vi "test Parse Sorted Object Dictionary_2.vi"(11 "Test Case In":refnum<class "test Electronic Datasheet.lvclass">) -> (0 "error out":errorcluster, 3 "Test Case Out":refnum<class "test Electronic Datasheet.lvclass">)   [LabVIEW 2024, in "test Electronic Datasheet.lvclass"]
uses:
  test Electronic Datasheet.lvclass
  C:/Program Files/National Instruments/LabVIEW 2024/vi.lib/Astemes/LUnit/Test Case.lvclass
  Core/Object Type.ctl
  Core/Access Type.ctl
  <vilib>/Astemes/LUnit/Test Case.lvclass/Test Case.ctl
  <vilib>/Astemes/LUnit/Append Fail Result.vi
  <vilib>/Astemes/LUnit/Append Pass Result.vi
  <vilib>/Astemes/LUnit/Run In UI.vi
  <vilib>/Utility/error.llb/Clear Errors.vi
  Core/OD Sub-Entry/OD Sub-Entry.lvclass
  D:/git/EDS-File-Viewer/Core/OD Entry/OD Entry.lvclass
  Electronic Datasheet/utils/Electronic Datasheet_GetAttributes.vi
  test Electronic Datasheet.lvclass/test Electronic Datasheet.ctl
  Electronic Datasheet/Electronic Datasheet.lvclass
  <vilib>/Astemes/LUnit/Test Case.lvclass
  Core/Electronic Datasheet.lvlib
  Core/OD Entry/OD Entry.lvclass
  D:/git/EDS-File-Viewer/Core/OD Sub-Entry/OD Sub-Entry.lvclass
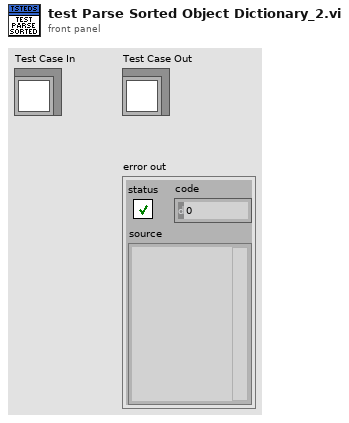
[diagram p1: front panel]
types:
  T1 = typedef "Electronic Datasheet.lvlib/Access Type.ctl" = enum16{"ro", "wo", "rw", "rwr", "rww", "const"}
  T2 = typedef "Electronic Datasheet.lvlib/Object Type.ctl" = u8
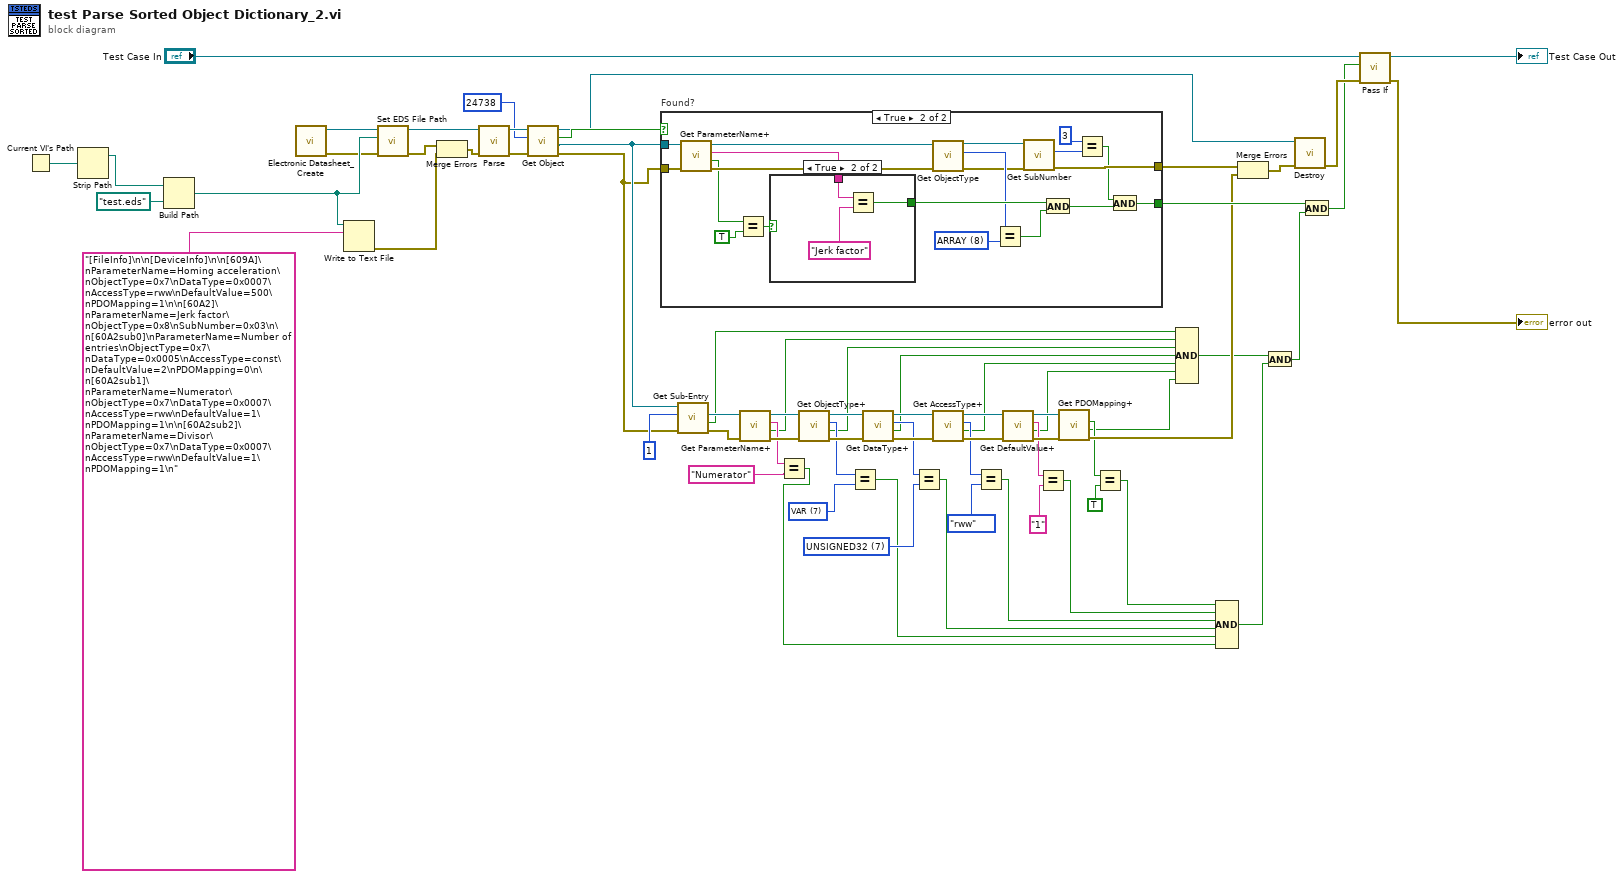
[diagram p0: block diagram]
diagram:
  w37 = u16 7 items=["BOOLEAN"=1, "INTEGER8"=2, "INTEGER16"=3, "INTEGER32"=4, "UNSIGNED8"=5, "UNSIGNED16"=6, "UNSIGNED32"=7, "REAL32"=8, "VISIBLE_STRING"=9, "OCTET_STRING"=10, "UNICODE_STRING"=11, "TIME_OF_DAY"=12, "TIME_DIFFERENCE"=13, "RESERVED1"=14, "DOMAIN"=15, "INTEGER24"=16, "REAL64"=17, "INTEGER40"=18, "INTEGER48"=19, "INTEGER56"=20, "INTEGER64"=21, "UNSIGNED24"=22, "RESERVED2"=23, "UNSIGNED40"=24, "UNSIGNED48"=25, "UNSIGNED56"=26, "UNSIGNED64"=27, "RESERVED3"=28, "RESERVED4"=29, "RESERVED5"=30, "RESERVED6"=31, "PDO_COMMUNICATION_PARAMETER"=32, "PDO_MAPPING"=33, "SDO_PARAMETER"=34, "IDENTITY"=35, "RESERVED7"=36] ("DataType")
  w39 = T2 7 items=["NULL"=0, "DOMAIN"=2, "DEFTYPE"=5, "DEFSTRUCT"=6, "VAR"=7, "ARRAY"=8, "RECORD"=9] ("ObjectType")
  n1 = Current VI's Path() -> (path=w64:path)
  n2 = Strip Path(path=w64) -> (stripped path=w60:path)  [unwired: 1 out]
  n3 = Build Path(base path=w60, name or relative path=path "test.eds") -> (appended path=w61:path)
  n4 = call "Electronic Datasheet_Create.vi"() -> ("Error Out"=w9:errorcluster, "reference out"=w10:refnum<class "Electronic Datasheet.lvclass">)  [unwired: 10 in]
  n5 = Write to Text File(file (use dialog)=w61, text="[FileInfo]\n\n[DeviceInfo]\n\n[609A]\nParameterName=Homing acceleration\nObjectType=0x7\nDataType=0x0007\nAccessType=rww\nDefaultValue=500\nPDOMapping=1\n\n[60A2]\nParameterName=Jerk factor\nObjectType=0x8\nSubNumber=0x03\n\n[60A2sub0]\nParameterName=Number of entries\nObjectType=0x7\nDataType=0x0005\nAccessType=const\nDefaultValue=2\nPDOMapping=0\n\n[60A2sub1]\nParameterName=Numerator\nObjectType=0x7\nDataType=0x0007\nAccessType=rww\nDefaultValue=1\nPDOMapping=1\n\n[60A2sub2]\nParameterName=Divisor\nObjectType=0x7\nDataType=0x0007\nAccessType=rww\nDefaultValue=1\nPDOMapping=1\n") -> (error out=w62:errorcluster)  [unwired: 2 in, 2 out]
  n6 = call "Set EDS File Path.vi"("error in"=w9, "EDS File Path"=w61, "reference in"=w10) -> ("error out"=w1:errorcluster, "reference out"=w65:refnum<class "Electronic Datasheet.lvclass">)  [unwired: 7 in]
  n7 = Merge Errors(w1, w62) -> (w2:errorcluster)
  n8 = call "Parse.vi"("error in"=w2, "reference in"=w65) -> ("error out"=w8:errorcluster, "reference out"=w59:refnum<class "Electronic Datasheet.lvclass">)  [unwired: 8 in]
  n9 = call "Get Object.vi"("error in"=w8, "Index"=u16 24738 ("Numeric"), "reference in"=w59) -> ("error out"=w4:errorcluster, "OD Entry"=w6:refnum<class "OD Entry.lvclass">, "Found?"=w5:bool, "reference out"=w3:refnum<class "Electronic Datasheet.lvclass">)  [unwired: 5 in]
  n10 = case "Found?" shown="True" w5 {
    selector: w5 -> [w69 _]
    tunnel: w6 -> [_ w90]
    tunnel: w4 -> [w70 w89]
    tunnel: [w69 w73] -> w57
    tunnel: [w70 w77] -> w55
    frame False {
    }
    frame True {
      w81 = T2 8 items=["NULL"=0, "DOMAIN"=2, "DEFTYPE"=5, "DEFSTRUCT"=6, "VAR"=7, "ARRAY"=8, "RECORD"=9] ("y")
      n11 = call "Get ParameterName+.vi"("Error In"=w89, "reference in"=w90) -> ("Error Out"=w83:errorcluster, "Defined?"=w71:bool, "ParameterName"=w87:string, "reference out"=w84:refnum<class "OD Entry.lvclass">)  [unwired: 6 in]
      n12 = Equal?(x=w71, y=TRUE) -> (x = y?=w86:bool)
      n13 = case shown="True" w86 {
        selector: w86 -> [w91 _]
        tunnel: w87 -> [_ w94]
        tunnel: [w91 w92] -> w85
        frame False {
        }
        frame True {
          n14 = Equal?(x=w94, y="Jerk factor") -> (x = y?=w92:bool)
        }
      }
      n15 = call "Get ObjectType.vi"("Error In"=w83, "reference in"=w84) -> ("Error Out"=w78:errorcluster, "ObjectType"=w82:T2, "reference out"=w76:refnum<class "OD Entry.lvclass">)  [unwired: 7 in]
      n16 = Equal?(x=w82, y=w81) -> (x = y?=w79:bool)
      n17 = call "Get SubNumber.vi"("Error In"=w78, "reference in"=w76) -> ("Error Out"=w77:errorcluster, "SubNumber"=w75:u8)  [unwired: 7 in, 1 out]
      n18 = And(x=w85, y=w79) -> (x .and. y?=w80:bool)
      n19 = Equal?(x=u8 3, y=w75) -> (x = y?=w72:bool)
      n20 = And(x=w72, y=w80) -> (x .and. y?=w73:bool)
    }
  }
  n21 = call "Get Sub-Entry.vi"("Error In"=w4, "Sub-Index"=u16 1, "reference in"=w6) -> ("Error Out"=w53:errorcluster, "Found?"=w41:bool, "OD Sub-Entry"=w54:refnum<class "OD Sub-Entry.lvclass">)  [unwired: 5 in, 1 out]
  n22 = call "Get ParameterName+.vi"("Error In"=w53, "reference in"=w54) -> ("Error Out"=w52:errorcluster, "Defined?"=w16:bool, "ParameterName"=w43:string, "reference out"=w51:refnum<class "OD Sub-Entry.lvclass">)  [unwired: 6 in]
  n23 = Equal?(x=w43, y="Numerator") -> (x = y?=w22:bool)
  n24 = call "Get ObjectType+.vi"("Error In"=w52, "reference in"=w51) -> ("Error Out"=w49:errorcluster, "Defined?"=w15:bool, "ObjectType"=w40:T2, "reference out"=w50:refnum<class "OD Sub-Entry.lvclass">)  [unwired: 6 in]
  n25 = Equal?(x=w40, y=w39) -> (x = y?=w21:bool)
  n26 = call "Get DataType+.vi"("Error In"=w49, "reference in"=w50) -> ("Error Out"=w46:errorcluster, "Defined?"=w14:bool, "DataType"=w38:u16, "reference out"=w47:refnum<class "OD Sub-Entry.lvclass">)  [unwired: 6 in]
  n27 = Equal?(x=w38, y=w37) -> (x = y?=w20:bool)
  n28 = call "Get AccessType+.vi"("Error In"=w46, "reference in"=w47) -> ("Error Out"=w44:errorcluster, "Defined?"=w13:bool, "AccessType"=w36:T1, "reference out"=w45:refnum<class "OD Sub-Entry.lvclass">)  [unwired: 6 in]
  n29 = Equal?(x=w36, y=Access_Type."rww") -> (x = y?=w19:bool)
  n30 = call "Get DefaultValue+.vi"("Error In"=w44, "reference in"=w45) -> ("Error Out"=w33:errorcluster, "Defined?"=w12:bool, "DefaultValue"=w31:string, "reference out"=w34:refnum<class "OD Sub-Entry.lvclass">)  [unwired: 6 in]
  n31 = Equal?(x=w31, y="1") -> (x = y?=w18:bool)
  n32 = call "Get PDOMapping+.vi"("Error In"=w33, "reference in"=w34) -> ("Error Out"=w32:errorcluster, "Defined?"=w11:bool, "PDOMapping"=w29:bool)  [unwired: 6 in, 1 out]
  n33 = Equal?(x=w29, y=TRUE) -> (x = y?=w17:bool)
  n34 = Compound Arithmetic op=AND(w41, w16, w15, w14, w13, w12, w11) -> (w25:bool)
  n35 = Compound Arithmetic op=AND(w17, w18, w19, w20, w21, w22) -> (w23:bool)
  n36 = Merge Errors(w55, w32) -> (w27:errorcluster)
  n37 = And(x=w25, y=w23) -> (x .and. y?=w24:bool)
  n38 = call-dynamic "Destroy.vi"("Error In"=w27, "reference in"=w3) -> ("Error Out"=w56:errorcluster)  [unwired: 8 in, 1 out]
  n39 = And(x=w57, y=w24) -> (x .and. y?=w26:bool)
  n40 = call <vilib>:"Pass If.vi"("error in (no error)"=w56, "Pass?"=w26, "LUnit Test Case In"="Test Case In") -> ("error out"=→"error out":errorcluster, "LUnit Test Case Out"=→"Test Case Out":refnum<class "test Electronic Datasheet.lvclass">)  [unwired: 7 in]
